vi "Set Child VI Ref.vi"(8 "error in (no error)":errorcluster, 9 "VI ref":refnum<vi>, 10 "Name":string, 11 "ActorMeter in":refnum<class "ActorMeter.lvclass">) -> (0 "error out":errorcluster, 3 "ActorMeter out":refnum<class "ActorMeter.lvclass">)   [LabVIEW 2014, in "ActorMeter.lvclass"]
uses:
  ActorMeter.lvclass
  ActorMeter.lvclass/ActorMeter.ctl
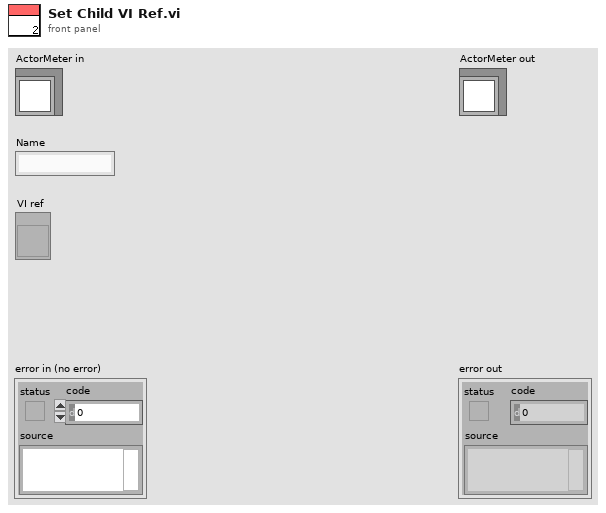
[diagram p1: front panel]
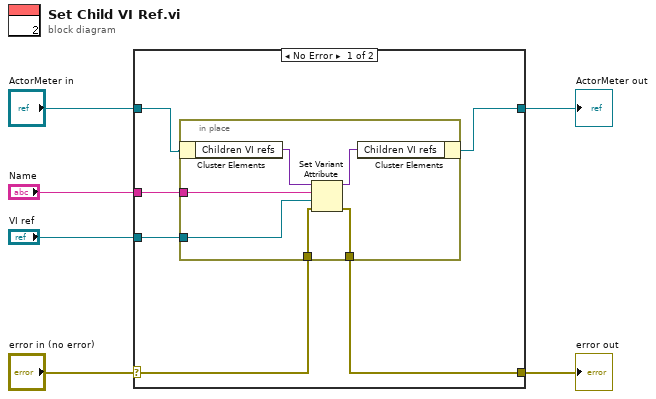
[diagram p0: block diagram]
diagram:
  n1 = case shown="No Error" "error in (no error)" {
    selector: "error in (no error)" -> [w10 w20]
    tunnel: [w9 w20] -> w5
    tunnel: [w7 w19] -> w3
    tunnel: "ActorMeter in" -> [w8 w19]
    tunnel: "Name" -> [w12 _]
    tunnel: "VI ref" -> [w11 _]
    frame No Error {
      n2 = in-place {
        in-place-border: w12 -> [w18]
        in-place-border: w11 -> [w17]
        in-place-border: w10 -> [w16]
        in-place-border: [w15] -> w9
        n3 = in-place-cluster #1(w8) -> ("Children VI refs"=w14:variant)
        n4 = Set Variant Attribute(Variant=w14, name=w18, value=w17, error in=w16) -> (Variant out=w13:variant, error out=w15:errorcluster)  [unwired: 1 out]
        n5 = in-place-cluster #1("Children VI refs"=w13) -> (w7:refnum<class "ActorMeter.lvclass">)
      }
    }
    frame Error {
    }
  }
  "error out" <- w5
  "ActorMeter out" <- w3
